vi "EEPROM StringToDate.vi"(8 "error in (no error)":errorcluster, 9 "Date String":string) -> (0 "error out":errorcluster, 1 "Date":string)   [LabVIEW 2010, in "lib1299.lvlib"]
doc: "XXX YYY"
uses:
  lib1299.lvlib
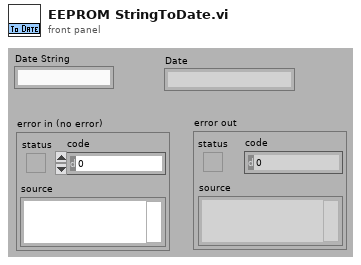
[diagram p1: front panel]
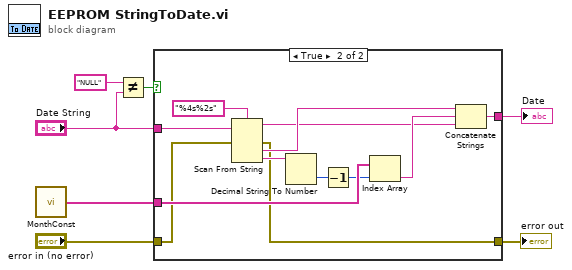
[diagram p0: block diagram]
diagram:
  n1 = call "MonthConst.vi"() -> ("Array"=w6:string[])  [unwired: 1 in]
  n2 = Not Equal?(x="NULL", y="Date String") -> (x != y?=w1:bool)
  n3 = case shown="True" w1 {
    tunnel: [w9 w20] -> w7
    tunnel: w6 -> [_ w15]
    tunnel: "error in (no error)" -> [w8 w12]
    tunnel: [w8 w11] -> w4
    tunnel: "Date String" -> [w9 w10]
    frame False {
    }
    frame True {
      n4 = Scan From String(format string="%4s%2s", input string=w10, error in=w12) -> (remaining string=w16:string, error out=w11:errorcluster, output 1=w18:string, output 2=w21:string)  [unwired: 3 in, 1 out]
      n5 = Decimal String To Number(string=w21) -> (number=w14:i32)  [unwired: 2 in, 1 out]
      n6 = Decrement(x=w14) -> (x-1=w13:i32)
      n7 = Index Array(array=w15, index=w13) -> (element=w17:string)
      n8 = Concatenate Strings(w18, w17, w16) -> (w20:string)
    }
  }
  "Date" <- w7
  "error out" <- w4
